vi "端口0.vi"(8 "数组 4":bool[](array[boolean]), 9 "数组 3":bool[](array[boolean]), 10 "数组 2":bool[](array[boolean]), 11 "数组":bool[](array[boolean])) -> ()   [LabVIEW 2018]
uses:
  <vilib>/rvi/eio/common/nirviEmuTemplateMethod_errors.vi
  <vilib>/eio/EIONode/EIONode.xnode
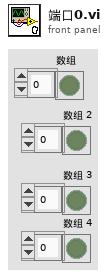
[diagram p1: front panel]
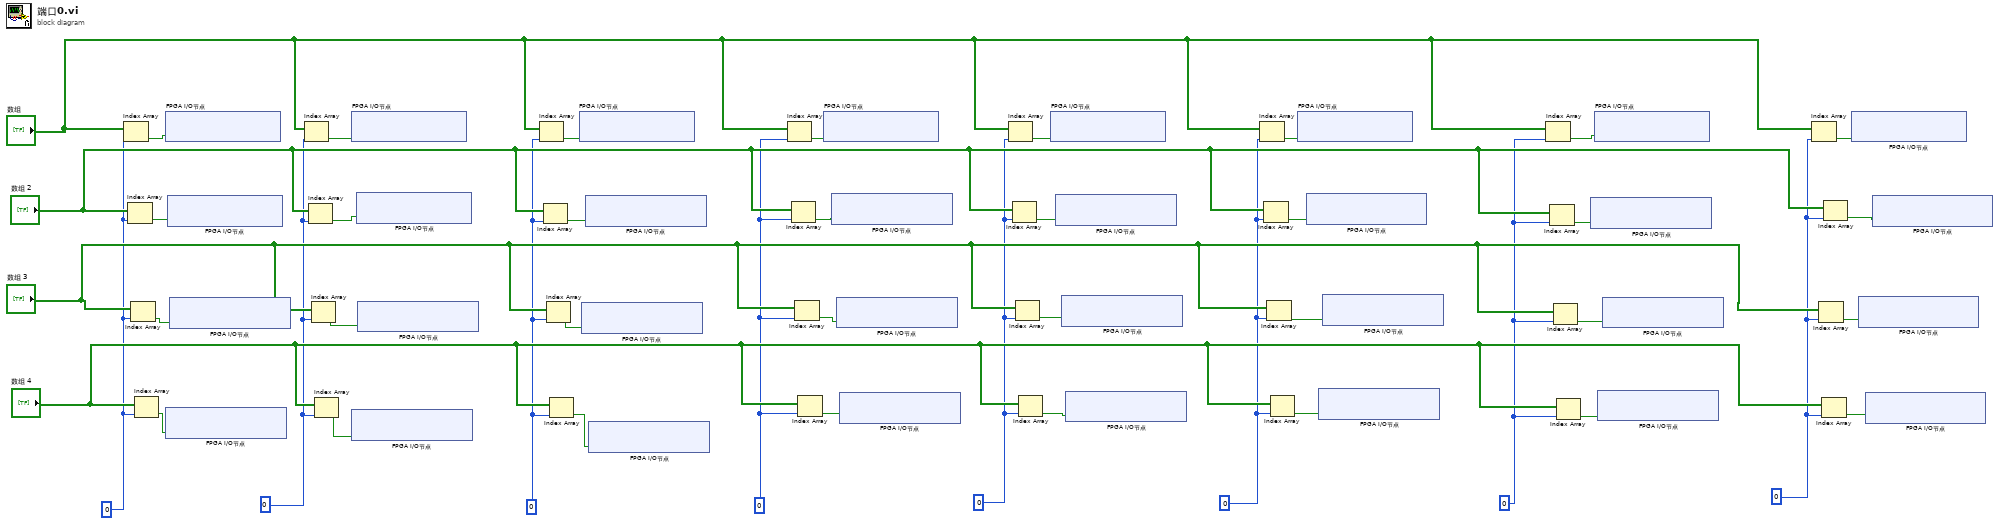
[diagram p0: block diagram]
diagram:
  w33 = i16 0
  w34 = i16 0
  w35 = i16 0
  w36 = i16 0
  w37 = i16 0
  w38 = i16 0
  w39 = i16 0
  w40 = i16 0
  n1 = Index Array(array="数组", index=w40) -> (element=w28:bool)
  n2 = Index Array(array="数组 2", index=w40) -> (element=w20:bool)
  n3 = Index Array(array="数组 3", index=w40) -> (element=w31:bool)
  n4 = Index Array(array="数组 4", index=w40) -> (element=w29:bool)
  n5 = xnode "FPGA I/O节点"("Connector0/DIO0"=w28) -> ()  [unwired: 1 in, 1 out]
  n6 = xnode "FPGA I/O节点"("Connector0/DIO24"=w29) -> ()  [unwired: 1 in, 1 out]
  n7 = xnode "FPGA I/O节点"("Connector0/DIO8"=w20) -> ()  [unwired: 1 in, 1 out]
  n8 = xnode "FPGA I/O节点"("Connector0/DIO16"=w31) -> ()  [unwired: 1 in, 1 out]
  n9 = Index Array(array="数组", index=w39) -> (element=w27:bool)
  n10 = Index Array(array="数组 2", index=w39) -> (element=w19:bool)
  n11 = Index Array(array="数组 3", index=w39) -> (element=w8:bool)
  n12 = Index Array(array="数组 4", index=w39) -> (element=w7:bool)
  n13 = xnode "FPGA I/O节点"("Connector0/DIO1"=w27) -> ()  [unwired: 1 in, 1 out]
  n14 = xnode "FPGA I/O节点"("Connector0/DIO25"=w7) -> ()  [unwired: 1 in, 1 out]
  n15 = xnode "FPGA I/O节点"("Connector0/DIO9"=w19) -> ()  [unwired: 1 in, 1 out]
  n16 = xnode "FPGA I/O节点"("Connector0/DIO17"=w8) -> ()  [unwired: 1 in, 1 out]
  n17 = Index Array(array="数组", index=w38) -> (element=w26:bool)
  n18 = Index Array(array="数组 2", index=w38) -> (element=w18:bool)
  n19 = Index Array(array="数组 3", index=w38) -> (element=w9:bool)
  n20 = Index Array(array="数组 4", index=w38) -> (element=w6:bool)
  n21 = xnode "FPGA I/O节点"("Connector0/DIO2"=w26) -> ()  [unwired: 1 in, 1 out]
  n22 = xnode "FPGA I/O节点"("Connector0/DIO18"=w9) -> ()  [unwired: 1 in, 1 out]
  n23 = xnode "FPGA I/O节点"("Connector0/DIO10"=w18) -> ()  [unwired: 1 in, 1 out]
  n24 = xnode "FPGA I/O节点"("Connector0/DIO26"=w6) -> ()  [unwired: 1 in, 1 out]
  n25 = Index Array(array="数组", index=w37) -> (element=w25:bool)
  n26 = Index Array(array="数组 2", index=w37) -> (element=w17:bool)
  n27 = Index Array(array="数组 3", index=w37) -> (element=w10:bool)
  n28 = Index Array(array="数组 4", index=w37) -> (element=w5:bool)
  n29 = xnode "FPGA I/O节点"("Connector0/DIO3"=w25) -> ()  [unwired: 1 in, 1 out]
  n30 = xnode "FPGA I/O节点"("Connector0/DIO11"=w17) -> ()  [unwired: 1 in, 1 out]
  n31 = xnode "FPGA I/O节点"("Connector0/DIO19"=w10) -> ()  [unwired: 1 in, 1 out]
  n32 = xnode "FPGA I/O节点"("Connector0/DIO27"=w5) -> ()  [unwired: 1 in, 1 out]
  n33 = Index Array(array="数组", index=w36) -> (element=w24:bool)
  n34 = Index Array(array="数组 2", index=w36) -> (element=w16:bool)
  n35 = Index Array(array="数组 3", index=w36) -> (element=w11:bool)
  n36 = Index Array(array="数组 4", index=w36) -> (element=w4:bool)
  n37 = xnode "FPGA I/O节点"("Connector0/DIO4"=w24) -> ()  [unwired: 1 in, 1 out]
  n38 = xnode "FPGA I/O节点"("Connector0/DIO12"=w16) -> ()  [unwired: 1 in, 1 out]
  n39 = xnode "FPGA I/O节点"("Connector0/DIO20"=w11) -> ()  [unwired: 1 in, 1 out]
  n40 = xnode "FPGA I/O节点"("Connector0/DIO28"=w4) -> ()  [unwired: 1 in, 1 out]
  n41 = Index Array(array="数组", index=w35) -> (element=w23:bool)
  n42 = Index Array(array="数组 2", index=w35) -> (element=w15:bool)
  n43 = Index Array(array="数组 3", index=w35) -> (element=w12:bool)
  n44 = Index Array(array="数组 4", index=w35) -> (element=w3:bool)
  n45 = xnode "FPGA I/O节点"("Connector0/DIO5"=w23) -> ()  [unwired: 1 in, 1 out]
  n46 = xnode "FPGA I/O节点"("Connector0/DIO13"=w15) -> ()  [unwired: 1 in, 1 out]
  n47 = xnode "FPGA I/O节点"("Connector0/DIO29"=w3) -> ()  [unwired: 1 in, 1 out]
  n48 = xnode "FPGA I/O节点"("Connector0/DIO21"=w12) -> ()  [unwired: 1 in, 1 out]
  n49 = Index Array(array="数组", index=w34) -> (element=w22:bool)
  n50 = Index Array(array="数组 2", index=w34) -> (element=w32:bool)
  n51 = Index Array(array="数组 3", index=w34) -> (element=w13:bool)
  n52 = Index Array(array="数组 4", index=w34) -> (element=w2:bool)
  n53 = xnode "FPGA I/O节点"("Connector0/DIO14"=w32) -> ()  [unwired: 1 in, 1 out]
  n54 = xnode "FPGA I/O节点"("Connector0/DIO6"=w22) -> ()  [unwired: 1 in, 1 out]
  n55 = xnode "FPGA I/O节点"("Connector0/DIO30"=w2) -> ()  [unwired: 1 in, 1 out]
  n56 = xnode "FPGA I/O节点"("Connector0/DIO22"=w13) -> ()  [unwired: 1 in, 1 out]
  n57 = Index Array(array="数组", index=w33) -> (element=w21:bool)
  n58 = Index Array(array="数组 3", index=w33) -> (element=w30:bool)
  n59 = Index Array(array="数组 4", index=w33) -> (element=w1:bool)
  n60 = Index Array(array="数组 2", index=w33) -> (element=w14:bool)
  n61 = xnode "FPGA I/O节点"("Connector0/DIO7"=w21) -> ()  [unwired: 1 in, 1 out]
  n62 = xnode "FPGA I/O节点"("Connector0/DIO23"=w30) -> ()  [unwired: 1 in, 1 out]
  n63 = xnode "FPGA I/O节点"("Connector0/DIO31"=w1) -> ()  [unwired: 1 in, 1 out]
  n64 = xnode "FPGA I/O节点"("Connector0/DIO15"=w14) -> ()  [unwired: 1 in, 1 out]
